vi "Create Session.vi"(5 "http-client (type)":refnum<class "http-client.lvclass">, 6 "verify server (true)":bool, 7 "cookie file":path, 8 "error in (no error)":errorcluster, 9 "password":string, 10 "username":string) -> (0 "error out":errorcluster, 3 "http-client out":refnum<class "http-client.lvclass">)   [LabVIEW 2020, in "http.lvlib" / "http-client.lvclass"]
uses:
  http-client.lvclass
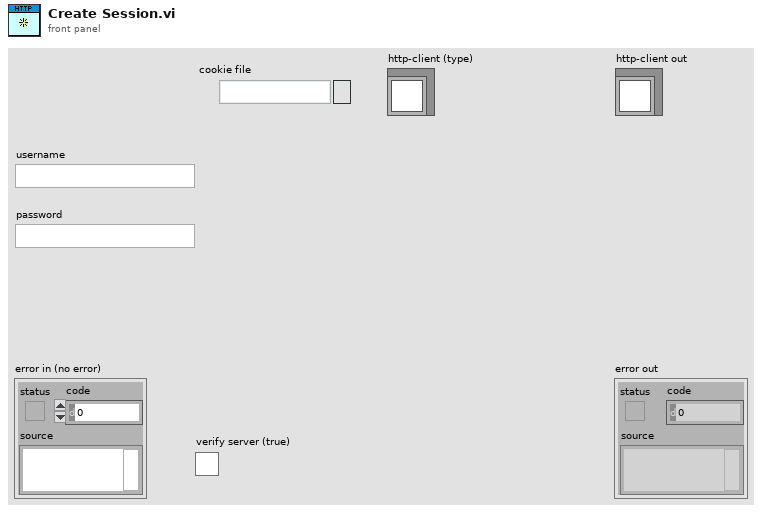
[diagram p1: front panel]
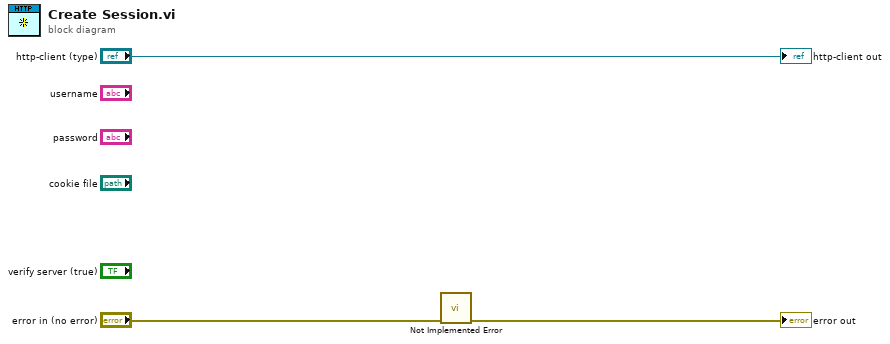
[diagram p0: block diagram]
diagram:
  n1 = call "Not Implemented Error.vi"("error in (no error)"="error in (no error)") -> ("error out"=→"error out":errorcluster)  [unwired: 10 in]
  "http-client out" <- "http-client (type)"
